vi "__goldopt_ab_x1x2.vi"(10 "bi":dbl, 11 "ai":dbl) -> (2 "x2":dbl, 3 "x1":dbl)   [LabVIEW 2017]
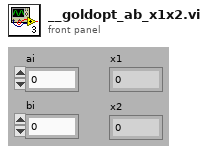
[diagram p1: front panel]
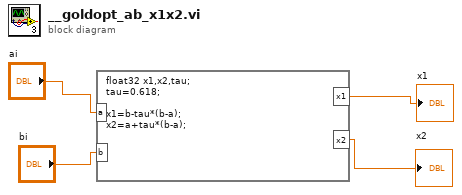
[diagram p0: block diagram]
diagram:
  n1 = formula code="float32 x1,x2,tau;\ntau=0.618;\n\nx1=b-tau*(b-a);\nx2=a+tau*(b-a);"("a"="ai", "b"="bi") -> ("x1"=→"x1":sgl, "x2"=→"x2":sgl)
